vi "ParseError.vi"(8 "error in (no error)":errorcluster, 11 "Microscope Controller in":refnum<class "MicroscopeController.lvclass">) -> (0 "error out":errorcluster, 3 "Microscope Controller out":refnum<class "MicroscopeController.lvclass">)   [LabVIEW 2020, in "MicroscopeController.lvlib" / "MicroscopeController.lvclass"]
uses:
  MicroscopeController.lvclass
  Model/Hardware Abstraction Layer/Component/Device/Device/DataExchange.ctl
  Interface/DataListener/DataListener.lvclass
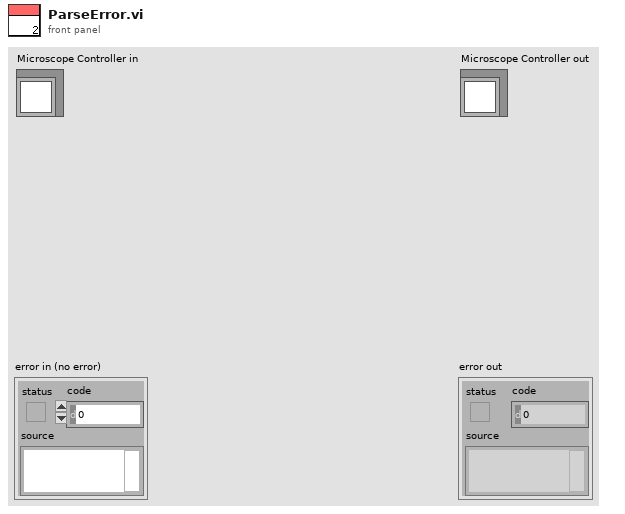
[diagram p1: front panel]
types:
  T1 = typedef "DataListener.lvclass/DataExchange.ctl" = cluster{"Source":string, "Destination":string, "Description":string, "value":variant}
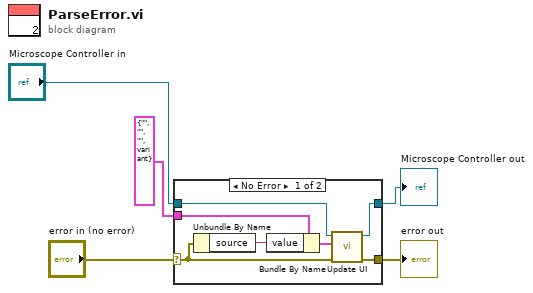
[diagram p0: block diagram]
diagram:
  n1 = case shown="No Error" "error in (no error)" {
    selector: "error in (no error)" -> [w8 w14]
    tunnel: T1 {"Source"="", "Destination"="", "Description"="", "value"=variant} ("DataExchange") -> [w12 _]
    tunnel: "Microscope Controller in" -> [w11 w13]
    tunnel: [w10 w14] -> w2
    tunnel: [w9 w13] -> w1
    frame No Error {
      n2 = Unbundle By Name(w8) -> ("source"=w6:string)
      n3 = Bundle By Name(cluster=w12, "value"=w6) -> (w7:T1)
      n4 = call "Update UI.vi"("error in (no error)"=w8, "DataExchange"=w7, "Microscope Controller in"=w11) -> ("error out"=w10:errorcluster, "Microscope Controller out"=w9:refnum<class "MicroscopeController.lvclass">)  [unwired: 7 in]
    }
    frame Error {
    }
  }
  "error out" <- w2
  "Microscope Controller out" <- w1
